vi "RunAvg.vi"(3 "Ignore avg?":bool, 5 "value in":dbl, 7 "# of samples":i32) -> (1 "value out":dbl)   [LabVIEW 2014]
panel:
  out "divisor":i32
  out "index":i32
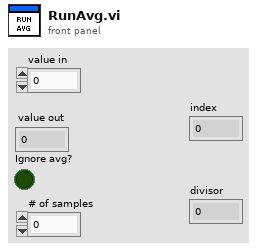
[diagram p1: front panel]
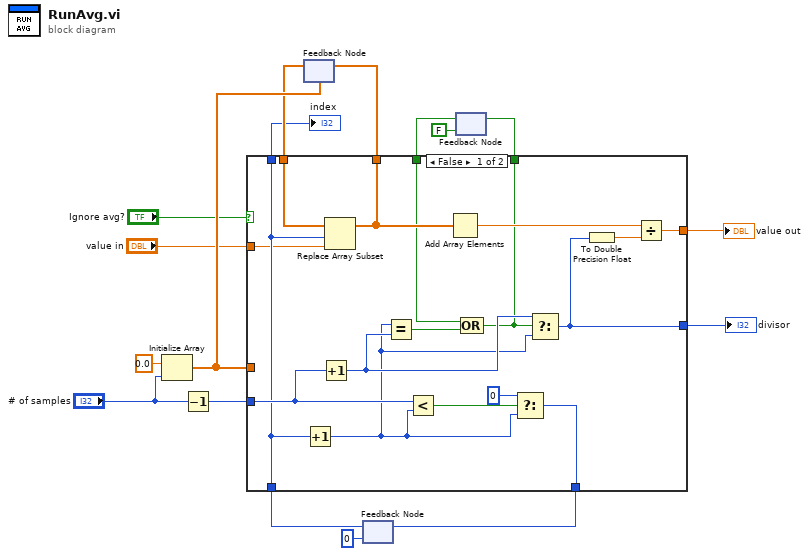
[diagram p0: block diagram]
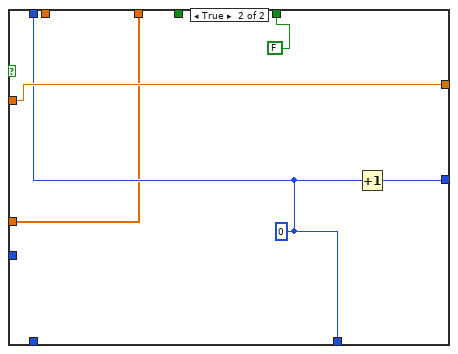
[diagram p2: hidden frame]
diagram:
  n1 = Initialize Array(0.0 ("element"), "# of samples") -> (w15:dbl[])
  n2 = Decrement(x="# of samples") -> (x-1=w12:i32)
  n3 = feedback #1(w15) -> (w14:dbl[])
  n4 = feedback #2(0 ("t")) -> (w11:i32)
  n5 = feedback #3(FALSE) -> (w3:bool)
  n6 = case shown="False" "Ignore avg?" {
    tunnel: w15 -> [_ w35]
    tunnel: w14 -> [w34 _]
    tunnel: [w33 w35] -> w13
    tunnel: w12 -> [w29 _]
    tunnel: w11 -> [w26 _]
    tunnel: [w27 w37] -> w10
    tunnel: [w26 w37] -> w8
    tunnel: [w23 w38] -> w7
    tunnel: [w22 w36] -> w6
    tunnel: [w21 FALSE] -> w5
    tunnel: w3 -> [w20 _]
    tunnel: "value in" -> [w19 w38]
    frame False {
      n7 = Increment(x=w26) -> (x+1=w18:i32)
      n8 = Increment(x=w29) -> (x+1=w30:i32)
      n9 = Replace Array Subset(array=w34, new element=w19, index=w26) -> (w33:dbl[])
      n10 = Equal?(x=w18, y=w30) -> (x = y?=w31:bool)
      n11 = Less?(x=w29, y=w18) -> (x < y?=w32:bool)
      n12 = Add Array Elements(numeric array=w33) -> (sum=w24:dbl)
      n13 = Compound Arithmetic op=OR(w20, w31) -> (w21:bool)
      n14 = Select(t=0, s=w32, f=w18) -> (s? t:f=w27:i32)
      n15 = Select(t=w30, s=w21, f=w18) -> (s? t:f=w22:i32)
      n16 = To Double Precision Float(number=w22) -> (double precision float=w25:dbl)
      n17 = Divide(x=w24, y=w25) -> (x/y=w23:dbl)
    }
    frame True {
      w37 = 0 ("x")
      n18 = Increment(x=w37) -> (x+1=w36:i32)
    }
  }
  "value out" <- w7
  "index" <- w8
  "divisor" <- w6
  n19 = feedback-in #1(w13) -> ()
  n20 = feedback-in #2(w10) -> ()
  n21 = feedback-in #3(w5) -> ()
